vi "Flatten.vi"(8 "error in (no error)":errorcluster, 11 "Varian Continuous in":refnum<class "Varian Continuous.lvclass">) -> (0 "error out":errorcluster, 3 "Varian Continuous out":refnum<class "Varian Continuous.lvclass">)   [LabVIEW 2009, in "Varian Continuous.lvclass"]
uses:
  Varian Continuous.lvclass
  Scanner/Scanner.lvclass
  Varian Continuous.lvclass/Varian Continuous.ctl
  Global/File Locations.vi
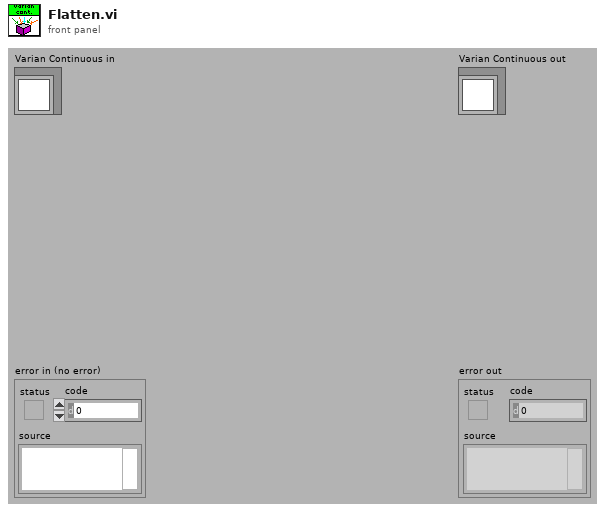
[diagram p1: front panel]
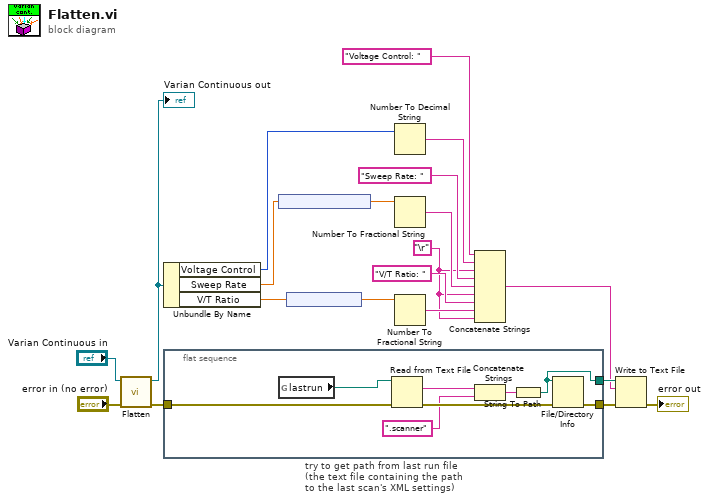
[diagram p0: block diagram]
diagram:
  w2 = "\r"
  n1 = call-parent "Flatten.vi"("error in (no error)"="error in (no error)", "Scanner in"="Varian Continuous in") -> ("error out"=w18:errorcluster, "Scanner out"=w14:refnum<class "Varian Continuous.lvclass">)  [unwired: 8 in]
  "Varian Continuous out" <- w14
  n2 = Unbundle By Name(w14) -> ("Voltage Control"=w9:u16, "Sweep Rate"=w12:dbl[unit], "V/T Ratio"=w13:dbl[unit])
  n3 = flat-sequence "try to get path from last run file\n(the text file containing the path\nto the last scan's XML settings)" {
    tunnel: [w28] -> w15
    tunnel: [w25] -> w16
    tunnel: w18 -> [w24]
    frame #0 {
      n4 = global read "File Locations.vi" "lastrun"() -> (w27:path)
      n5 = Read from Text File(file (use dialog)=w27, error in=w24) -> (text=w23:string, error out=w26:errorcluster)  [unwired: 4 out]
      n6 = Concatenate Strings(w23, ".scanner") -> (w21:string)
      n7 = String To Path(string=w21) -> (path=w28:path)
      n8 = File/Directory Info(path=w28, error in=w26) -> (error out=w25:errorcluster)  [unwired: 6 out]
    }
  }
  n9 = node(w12) -> (w10:dbl)
  n10 = node(w13) -> (w11:dbl)
  n11 = Number To Decimal String(number=w9) -> (decimal integer string=w8:string)  [unwired: 1 in]
  n12 = Number To Fractional String(number=w10) -> (F-format string=w5:string)  [unwired: 3 in]
  n13 = Number To Fractional String(number=w11) -> (F-format string=w3:string)  [unwired: 3 in]
  n14 = Concatenate Strings("Voltage Control: ", w8, w2, "Sweep Rate: ", w5, w2, "V/T Ratio: ", w3, w2) -> (w1:string)
  n15 = Write to Text File(file (use dialog)=w15, text=w1, error in=w16) -> (error out=→"error out":errorcluster)  [unwired: 1 in, 2 out]
